vi "PointCloudTesting.vi"() -> ()   [LabVIEW 2016]
uses:
  <vilib>/Utility/miscctls.llb/LVRGBAColorTypeDef.ctl
  <vilib>/Utility/miscctls.llb/LV3DPointTypeDef.ctl
  <vilib>/picture/3D Picture Control/Object/Create Object (name).vi
  <vilib>/picture/3D Picture Control/NI_3D Picture Control.lvlib
panel:
  in  "Color Binding Mode":T1(ring)=enum."Per Vertex"
  in  "file path (dialog if empty)":path
  in  "From File?":bool
  in  "Camera Controller:":T2(ring)=enum."Spherical"
  in  "stop":bool
  out "3D Picture":refnum<vi>(3d-picture)
  # "Overview:  Code that shows how to load a 3D point cloud data into a 3D picture control in LabVIEW.\nRequirements: LabVIEW 2012 or compatible\nInstructions:\n1. Select if you would like to load from file or generate a random object.\n2. Run the VI.\n3. Use the Camera Controller to adjust the way the mouse moves the 3D object."
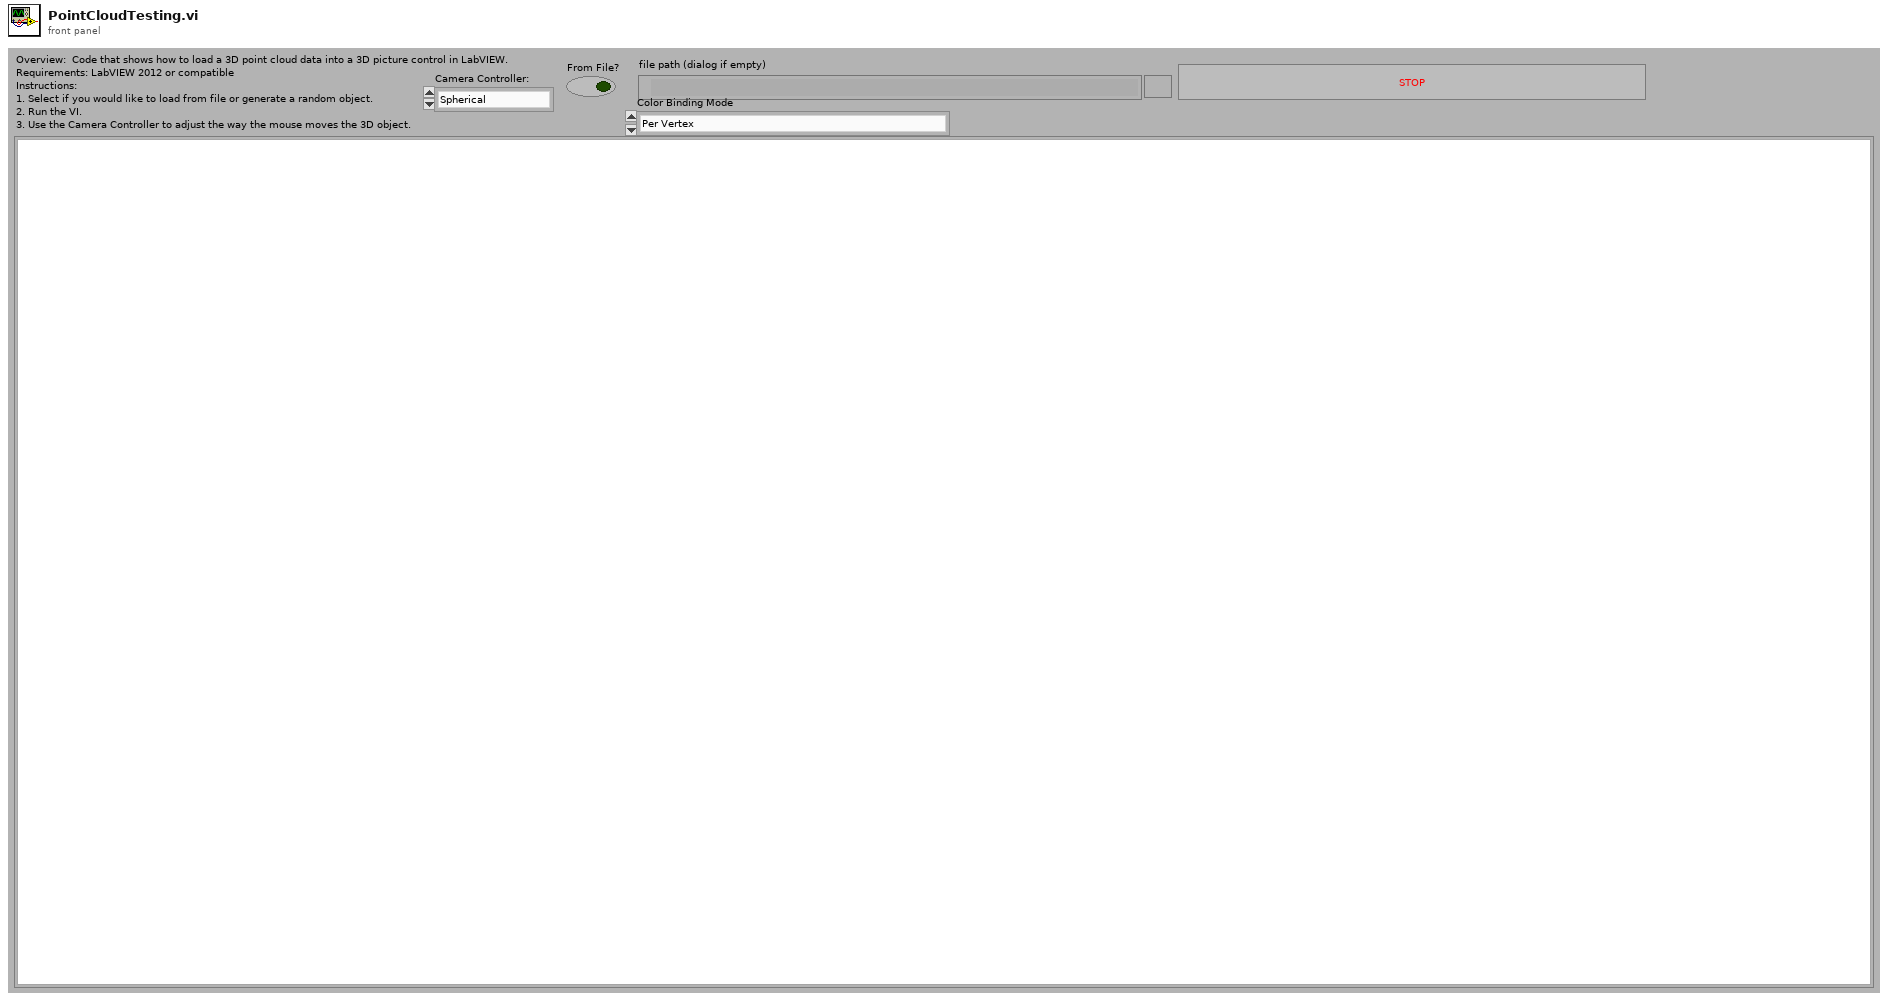
[diagram p1: front panel]
types:
  T1 = enum16{"Overall", "Per Primitive", "Per Vertex", "Binding Off"}
  T2 = enum16{"None", "Spherical", "Flying", "Oriented"}
  T3 = enum16{"Points", "Lines", "Line Strip", "Line Loop", "Triangles", "Triangle Strip", "Triangle Fan", "Quads", "Quad Strip", "Polygon"}
  T4 = typedef "LVRGBAColorTypeDef.ctl" = cluster{"Red":sgl, "Green":sgl, "Blue":sgl, "Alpha":sgl}
  T5 = typedef "LV3DPointTypeDef.ctl" = cluster{"X":sgl, "Y":sgl, "Z":sgl}
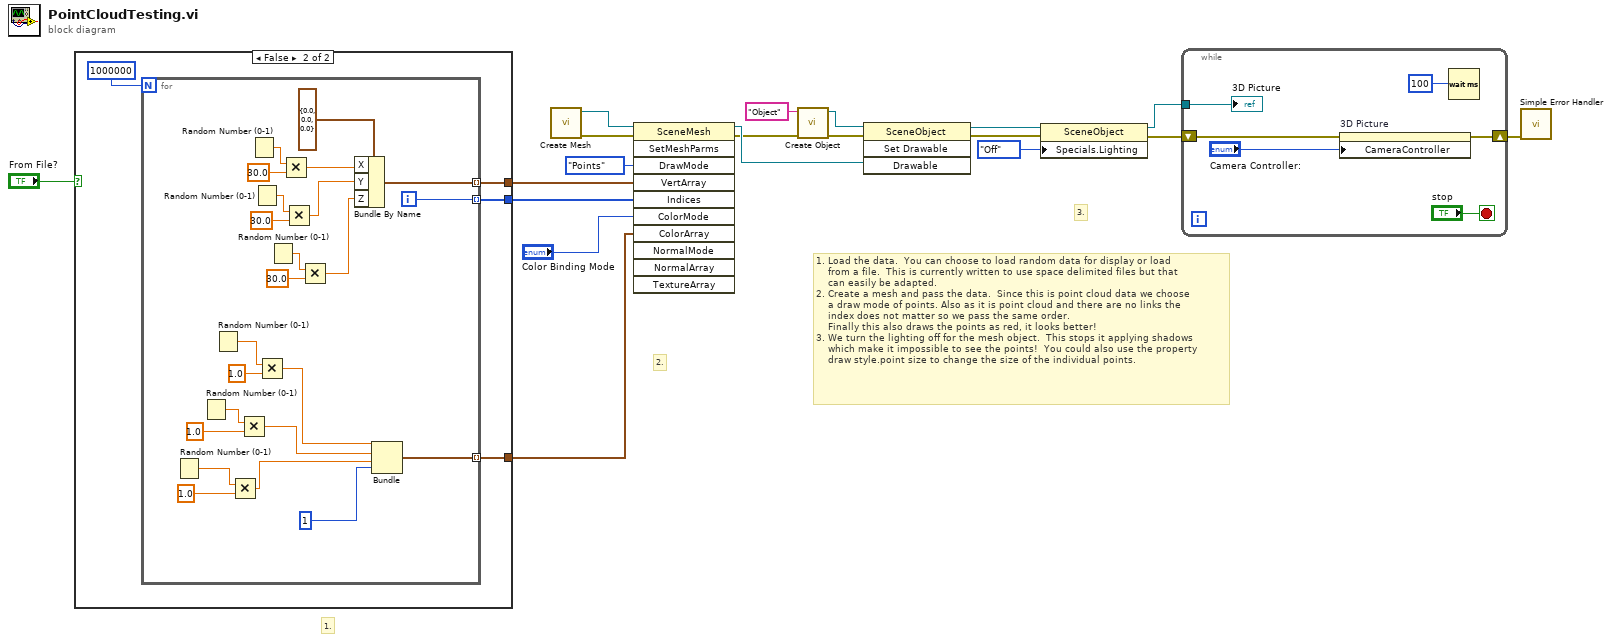
[diagram p0: block diagram]
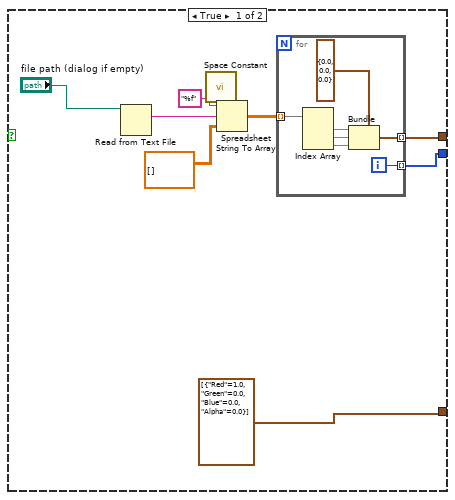
[diagram p2: hidden frame]
diagram:
  # "1. Load the data.  You can choose to load random data for display or load \n    from a file.  This is currently written to use space delimited files but that\n    can easily be adapted.\n2. Create a mesh and pass the data.  Since this is point cloud data we choose\n    a draw mode of points. Also as it is point cloud and there are no links the \n    index does not matter so we pass the same order.\n    Finally this also draws the points as red, it looks better!\n3. We turn the lighting off for the mesh object.  This stops it applying shadows\n    which make it impossible to see the points!  You could also use the property\n    draw style.point size to change the size of the individual points."
  # "3."
  # "2."
  # "1."
  n1 = case shown="False" "From File?" {
    tunnel: [w22 w38] -> w17
    tunnel: [w21 w37] -> w8
    tunnel: [T4[] [{"Red"=1.0, "Green"=0.0, "Blue"=0.0, "Alpha"=0.0}] w36] -> w1
    frame True {
      n2 = Read from Text File(file (use dialog)="file path (dialog if empty)") -> (text=w27:string)  [unwired: 3 in, 3 out]
      n3 = call <vilib>:"Space Constant.vi"() -> ("String"=w26:string)
      n4 = Spreadsheet String To Array(delimiter (Tab)=w26, format string="%f", spreadsheet string=w27, array type (2D Dbl)=sgl[][] []) -> (array=w24:sgl[][])
      n5 = for {
        tunnel: w24 -> [w35] mode=indexing
        tunnel: [w30] -> w22 mode=indexing
        tunnel: [w29] -> w21 mode=indexing
        i -> [w29]
        n6 = Index Array(array=w35) -> (element #1=w33:sgl, element #2=w32:sgl, element #3=w31:sgl)  [unwired: 3 in]
        n7 = Bundle(cluster=T5 {"X"=0.0, "Y"=0.0, "Z"=0.0} ("3D Point"), "X"=w33, "Y"=w32, "Z"=w31) -> (w30:T5)
      }
    }
    frame False {
      n8 = for {
        N: 1000000 -> [_]
        tunnel: [w52] -> w38 mode=indexing
        tunnel: [w51] -> w37 mode=indexing
        tunnel: [w42] -> w36 mode=indexing
        i -> [w51]
        n9 = Random Number (0-1)() -> (number: 0 to 1=w47:dbl)
        n10 = Random Number (0-1)() -> (number: 0 to 1=w40:dbl)
        n11 = Random Number (0-1)() -> (number: 0 to 1=w50:dbl)
        n12 = Multiply(x=w47, y=1.0) -> (x*y=w43:dbl)
        n13 = Multiply(x=w40, y=1.0) -> (x*y=w44:dbl)
        n14 = Random Number (0-1)() -> (number: 0 to 1=w60:dbl)
        n15 = Random Number (0-1)() -> (number: 0 to 1=w59:dbl)
        n16 = Multiply(x=w50, y=1.0) -> (x*y=w45:dbl)
        n17 = Random Number (0-1)() -> (number: 0 to 1=w56:dbl)
        n18 = Multiply(x=w60, y=30.0) -> (x*y=w55:dbl)
        n19 = Multiply(x=w59, y=30.0) -> (x*y=w54:dbl)
        n20 = Multiply(x=w56, y=30.0) -> (x*y=w53:dbl)
        n21 = Bundle By Name(cluster=T5 {"X"=0.0, "Y"=0.0, "Z"=0.0} ("3D Point"), "X"=w55, "Y"=w54, "Z"=w53) -> (w52:T5)
        n22 = Bundle(w45, w44, w43, 1) -> (w42:cluster{dbl, dbl, dbl, i32})  [unwired: 1 in]
      }
    }
  }
  n23 = call <vilib>:"Create Mesh.vi"() -> ("error out"=w7:errorcluster, "New Mesh Refnum"=w15:refnum<vi>)  [unwired: 10 in]
  n24 = invoke class="SceneMesh" method="SetMeshParms"(reference=w15, error in=w7, "DrawMode"=T3."Points" ("Draw Mode"), "VertArray"=w17, "Indices"=w8, "ColorMode"="Color Binding Mode", "ColorArray"=w1) -> (reference out=w12:refnum<vi>, error out=w4:errorcluster)  [unwired: 4 in, 9 out]
  n25 = call-poly <vilib>:"Create Object.vi"("error in (no error)"=w4, "Name"="Object") -> ("error out"=w3:errorcluster, "Scene:New Object"=w18:refnum<vi>)  [unwired: 8 in]
  n26 = invoke class="SceneObject" method="Set Drawable"(reference=w18, error in=w3, "Drawable"=w12) -> (reference out=w11:refnum<vi>, error out=w6:errorcluster)  [unwired: 1 in, 2 out]
  n27 = property class="SceneObject"(reference=w11, error in=w6, "Specials.Lighting"=enum16{"Inherit Value", "Off", "On"}."Off" ("Specials:Lighting")) -> (reference out=w10:refnum<vi>, error out=w5:errorcluster)
  n28 = while {
    tunnel: w10 -> [w68]
    shift-right: [w63] -> w2
    shift-left: w5 -> [w64]
    stop <- "stop" stop-if-true
    n29 = property on="3D Picture" class="SceneGraphDisp (strict)"(error in=w64, "CameraController"="Camera Controller:") -> (error out=w63:errorcluster)  [unwired: 1 in, 1 out]
    n30 = Wait (ms)(milliseconds to wait=u32 100 ("millisecond multiple")) -> ()  [unwired: 1 out]
    "3D Picture" <- w68
  }
  n31 = call <vilib>:"Simple Error Handler.vi"("error in (no error)"=w2) -> ()  [unwired: 4 in, 5 out]
